vi "Grave from Bookmark Label.vi"(8 "Error In":errorcluster, 10 "Bookmark ID":i32, 11 "VI In":refnum<vi>) -> (0 "Error Out":errorcluster, 2 "Grave":refnum<vi>, 3 "VI Out":refnum<vi>)   [LabVIEW 2018, in "Bookmark Manager.lvlib"]
uses:
  Bookmark Manager.lvlib
  <vilib>/Utility/traverseref.llb/TRef TravTarget.ctl
  <vilib>/Utility/traverseref.llb/VI Scripting - Traverse.lvlib
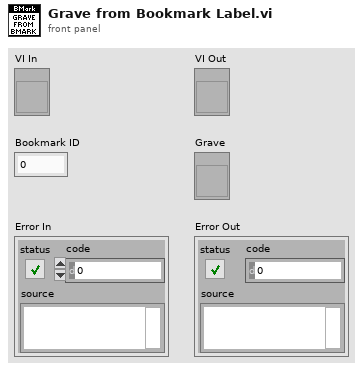
[diagram p1: front panel]
types:
  T1 = typedef "TRef TravTarget.ctl" = enum16{"FP", "BD", "Other"}
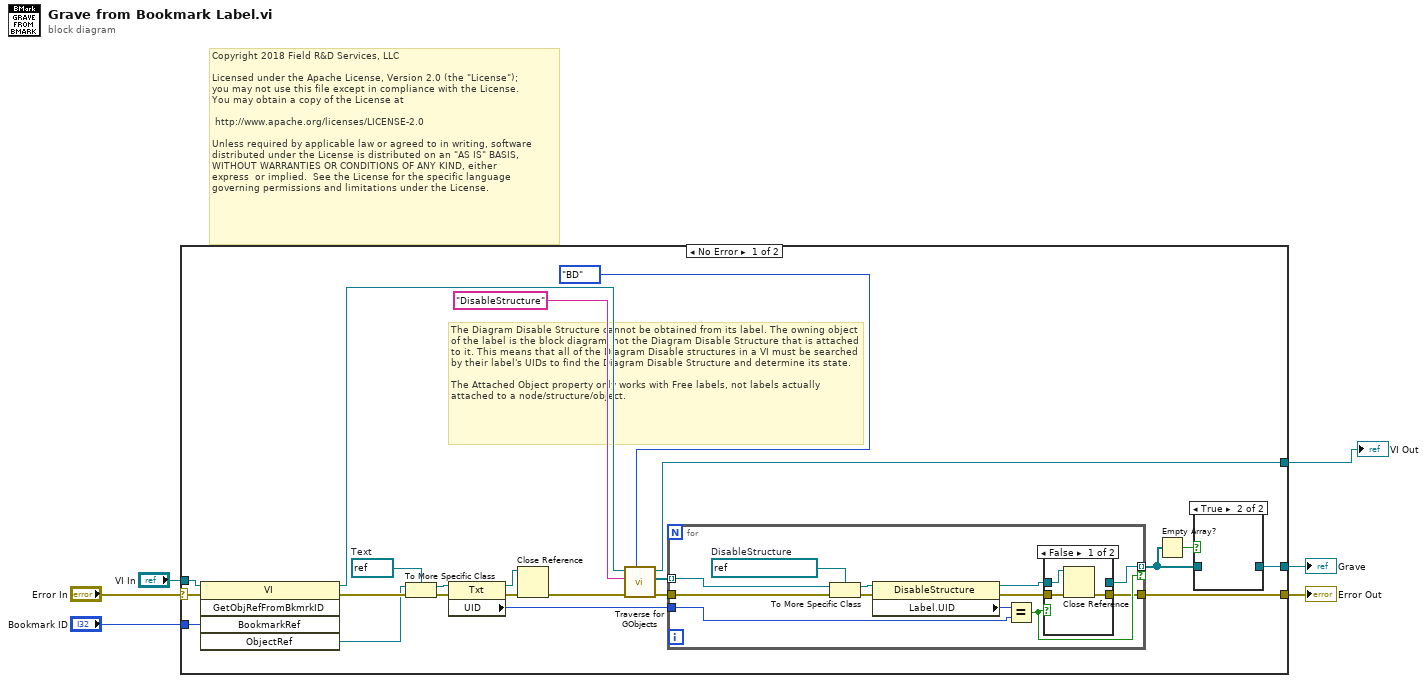
[diagram p0: block diagram]
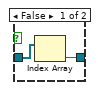
[diagram p2: hidden frame]
diagram:
  # "Copyright 2018 Field R&D Services, LLC\n\nLicensed under the Apache License, Version 2.0 (the \"License\");\nyou may not use this file except in compliance with the License.\nYou may obtain a copy of the License at\n\n\thttp://www.apache.org/licenses/LICENSE-2.0\n\nUnless required by applicable law or agreed to in writing, software\ndistributed under the License is distributed on an \"AS IS\" BASIS,\nWITHOUT WARRANTIES OR CONDITIONS OF ANY KIND, either \nexpress  or implied.  See the License for the specific language \ngoverning permissions and limitations under the License."
  n1 = case shown="No Error" "Error In" {
    selector: "Error In" -> [w8 w49]
    tunnel: [w18 w49] -> w6
    tunnel: [w14 _] -> w5
    tunnel: "VI In" -> [w13 w48]
    tunnel: "Bookmark ID" -> [w9 _]
    tunnel: [w7 w48] -> w1
    frame No Error {
      w24 = refnum<vi> refnum  # Text
      # "The Diagram Disable Structure cannot be obtained from its label. The owning object of the label is the block diagram, not the Diagram Disable Structure that is attached to it. This means that all of the Diagram Disable structures in a VI must be searched by their label's UIDs to find the Diagram Disable Structure and determine its state.\n\nThe Attached Object property only works with Free labels, not labels actually attached to a node/structure/object."
      n2 = invoke class="VI" method="GetObjRefFromBkmrkID"(reference=w13, error in=w8, "BookmarkRef"=w9) -> (reference out=w12:refnum<vi>, error out=w11:errorcluster, "ObjectRef"=w10:refnum<vi>)  [unwired: 2 in, 2 out]
      n3 = To More Specific Class(target class=w24, reference=w10, error in=w11) -> (specific class reference=w22:refnum<vi>, error out=w23:errorcluster)
      n4 = property class="Txt"(reference=w22, error in=w23) -> (reference out=w28:refnum<vi>, error out=w25:errorcluster, "UID"=w19:i32)
      n5 = Close Reference(reference=w28, error in (no error)=w25) -> (error out=w27:errorcluster)
      n6 = call <vilib>:"Traverse for GObjects.vi"("Traverse Target"=TRef_TravTarget."BD", "error in (no error)"=w27, "Class Name"="DisableStructure", "VI Refnum"=w12) -> ("error out"=w26:errorcluster, "References"=w17:refnum<vi>[], "dup VI Refnum"=w7:refnum<vi>)  [unwired: 4 in, 1 out]
      n7 = for {
        tunnel: w17 -> [w42] mode=indexing
        tunnel: w19 -> [w36]
        tunnel: w26 -> [w40]
        tunnel: [w33] -> w18
        tunnel: [w31] -> w15 mode=indexing if=w35
        w41 = refnum<vi> refnum  # DisableStructure
        n8 = To More Specific Class(target class=w41, reference=w42, error in=w40) -> (specific class reference=w38:refnum<vi>, error out=w39:errorcluster)
        n9 = property class="DisableStructure"(reference=w38, error in=w39) -> (reference out=w32:refnum<vi>, error out=w34:errorcluster, "Label.UID"=w37:i32)
        n10 = Equal?(x=w37, y=w36) -> (x = y?=w35:bool)
        n11 = case shown="False" w35 {
          tunnel: w34 -> [w45 w47]
          tunnel: [w44 w47] -> w33
          tunnel: w32 -> [w43 w46]
          tunnel: [_ w46] -> w31
          frame False {
            n12 = Close Reference(reference=w43, error in (no error)=w45) -> (error out=w44:errorcluster)
          }
          frame True {
          }
        }
      }
      n13 = Empty Array?(array=w15) -> (empty?=w16:bool)
      n14 = case shown="True" w16 {
        tunnel: w15 -> [w30 _]
        tunnel: [w29 _] -> w14
        frame False {
          n15 = Index Array(array=w30) -> (element=w29:refnum<vi>)  [unwired: 1 in]
        }
        frame True {
        }
      }
    }
    frame Error {
    }
  }
  "Error Out" <- w6
  "Grave" <- w5
  "VI Out" <- w1
